vi "ImageAlreadyProcessed.vi"(1 "Array":i32[](array[numeric]), 2 "Numeric":i32, 3 "subscriber list":string) -> (0 "Boolean":bool)   [LabVIEW 2013]
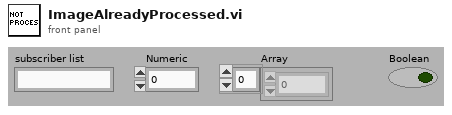
[diagram p1: front panel]
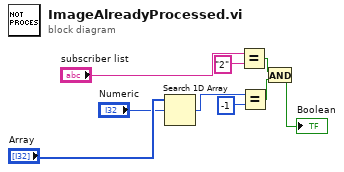
[diagram p0: block diagram]
diagram:
  n1 = Search 1D Array(1D array="Array", element="Numeric") -> (index of element=w4:i32)  [unwired: 1 in]
  n2 = Equal?(x="subscriber list", y="2") -> (x = y?=w6:bool)
  n3 = Equal?(x=w4, y=-1) -> (x = y?=w7:bool)
  n4 = And(x=w6, y=w7) -> (x .and. y?=→"Boolean":bool)
